vi "Copy to Matching Items.vi"(9 "Front Panel Controls":T1, 11 "Item Data":refnum<class "Item.lvclass">[](array[class])) -> (3 "Item Data out":refnum<class "Item.lvclass">[](array[class]))   [LabVIEW 2020, in "VI Properties Editor.lvlib"]
doc: "Copies current VI properties to all VIs whose name matches the one currently being edited."
uses:
  VI Properties Editor.lvlib
  Classes/Item/Item.lvclass
  CTLs/Main Front Panel Controls.ctl
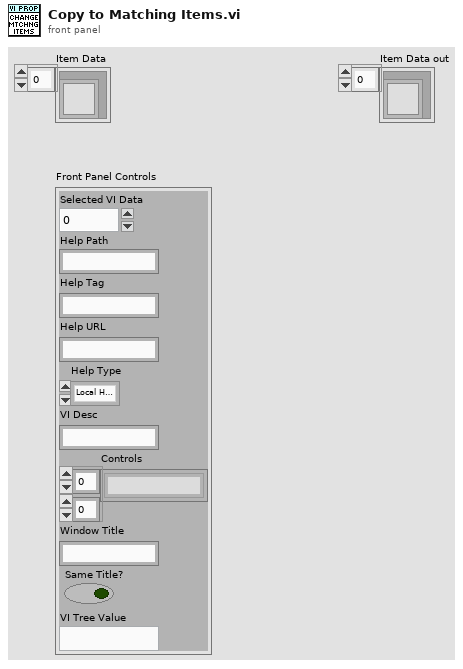
[diagram p1: front panel]
types:
  T1 = typedef "VI Properties Editor.lvlib/Main Front Panel Controls.ctl" = cluster{"Selected VI Data":i32, "Help Path":string, "Help Tag":string, "Help URL":string, "Help Type":enum16{"Local Help File", "Web-based Help"}, "VI Desc":string, "Controls":string[][], "Window Title":string, "Same Title?":bool, "VI Tree Value":string}
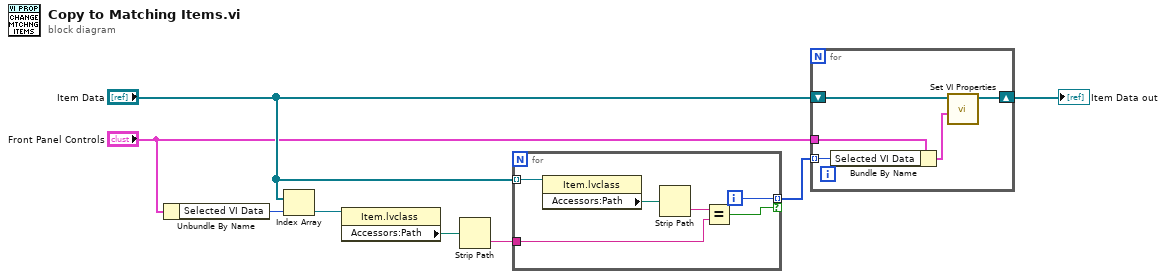
[diagram p0: block diagram]
diagram:
  n1 = Unbundle By Name("Front Panel Controls") -> ("Selected VI Data"=w5:i32)
  n2 = Index Array(array="Item Data", index=w5) -> (element=w2:refnum<class "Item.lvclass">)
  n3 = property class="Item.lvclass"(reference=w2) -> ("Accessors:Path"=w1:path)  [unwired: 1 in, 2 out]
  n4 = Strip Path(path=w1) -> (name=w4:string)  [unwired: 1 out]
  n5 = for {
    tunnel: "Item Data" -> [w10] mode=indexing
    tunnel: w4 -> [w14]
    tunnel: [w12] -> w7 mode=indexing if=w11
    i -> [w12]
    n6 = property class="Item.lvclass"(reference=w10) -> ("Accessors:Path"=w9:path)  [unwired: 1 in, 2 out]
    n7 = Strip Path(path=w9) -> (name=w13:string)  [unwired: 1 out]
    n8 = Equal?(x=w13, y=w14) -> (x = y?=w11:bool)
  }
  n9 = for {
    tunnel: w7 -> [w16] mode=indexing
    shift-right: [w15] -> w8
    shift-left: "Item Data" -> [w19]
    tunnel: "Front Panel Controls" -> [w18]
    n10 = Bundle By Name(cluster=w18, "Selected VI Data"=w16) -> (w17:T1)
    n11 = call "Set VI Properties.vi"("Front Panel Controls"=w17, "Item Data"=w19) -> ("Item Data out"=w15:refnum<class "Item.lvclass">[])  [unwired: 9 in]
  }
  "Item Data out" <- w8
